vi "PreExplorer.vi"(10 "Application Directory":path, 11 ".NET 참조 번호 입력":refnum<k24>) -> (0 "에러 출력":errorcluster, 3 ".NET 참조 번호 출력":refnum<k24>)   [LabVIEW 2017, in "Retrieved Data.lvclass"]
uses:
  Retrieved Data.lvclass
  C:/Users/KimYG/Application/Solution Package/Minhee Retriever/binaries/Microsoft.WindowsAPICodePack.Shell.dll
  binaries/Microsoft.WindowsAPICodePack.Shell.dll
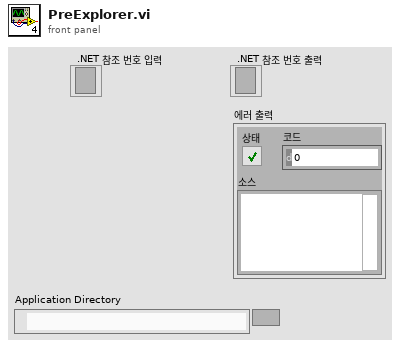
[diagram p1: front panel]
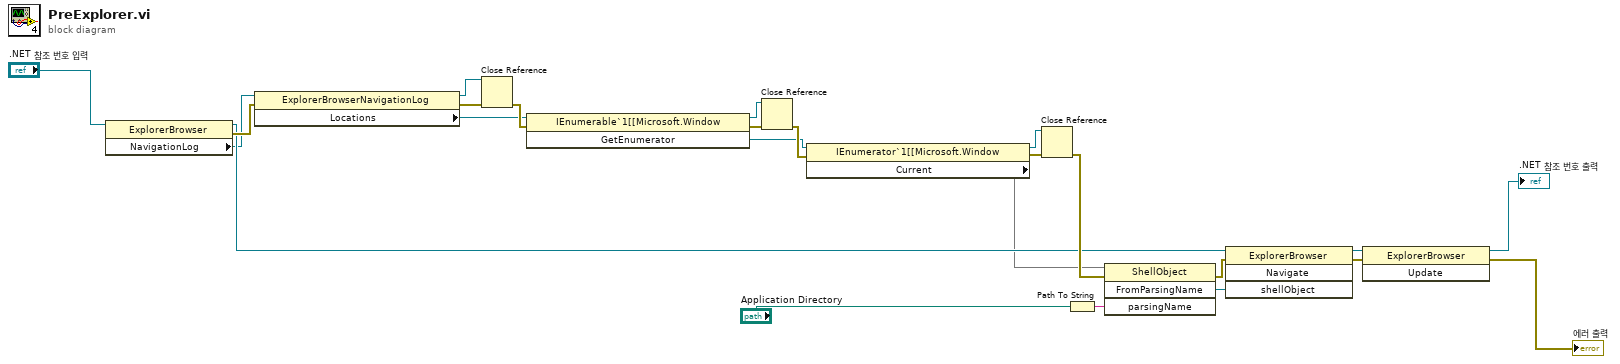
[diagram p0: block diagram]
diagram:
  n1 = property class="ExplorerBrowser"(reference=".NET 참조 번호 입력") -> (reference out=w8:refnum<k24>, error out=w12:errorcluster, "NavigationLog"=w1:refnum<k24>)  [unwired: 1 in]
  n2 = property class="ExplorerBrowserNavigationLog"(reference=w1, error in=w12) -> (reference out=w22:refnum<k24>, error out=w23:errorcluster, "Locations"=w5:refnum<k24>)
  n3 = Close Reference(reference=w22, error in (no error)=w23) -> (error out=w24:errorcluster)
  n4 = invoke class="IEnumerable`1[[Microsoft.Window" method="GetEnumerator"(reference=w5, error in=w24) -> (reference out=w20:refnum<k24>, error out=w19:errorcluster, "GetEnumerator"=w6:refnum<k24>)  [unwired: 1 in]
  n5 = Close Reference(reference=w20, error in (no error)=w19) -> (error out=w21:errorcluster)
  n6 = property class="IEnumerator`1[[Microsoft.Window"(reference=w6, error in=w21) -> (reference out=w17:refnum<k24>, error out=w16:errorcluster, "Current"=w2)
  n7 = Close Reference(reference=w17, error in (no error)=w16) -> (error out=w18:errorcluster)
  n8 = Path To String(path="Application Directory") -> (string=w15:string)
  n9 = invoke class="ShellObject" method="FromParsingName"(reference=w2, error in=w18, "parsingName"=w15) -> (error out=w11:errorcluster, "FromParsingName"=w3:refnum<k24>)  [unwired: 1 in, 2 out]
  n10 = invoke class="ExplorerBrowser" method="Navigate"(reference=w8, error in=w11, "shellObject"=w3) -> (reference out=w13:refnum<k24>, error out=w4:errorcluster)  [unwired: 1 in, 2 out]
  n11 = invoke class="ExplorerBrowser" method="Update"(reference=w13, error in=w4) -> (reference out=→".NET 참조 번호 출력":refnum<k24>, error out=→"에러 출력":errorcluster)  [unwired: 1 in, 1 out]
